vi "PH_PP_CurrentMeas.stop Task.vi"(0 "i ref in":refnum<vi>, 2 "Task #":i32, 5 "error in (no error)":errorcluster) -> (14 "i ref out":refnum<vi>, 19 "error out":errorcluster)   [LabVIEW 2014, in "PH_PP_CurrentMeas.lvlib"]
uses:
  PH_PP_CurrentMeas.lvlib
  PH_StatusHandler/PH_StatusHandler.Status.ctl
  PH_StatusHandler/PH_StatusHandler.lvlib
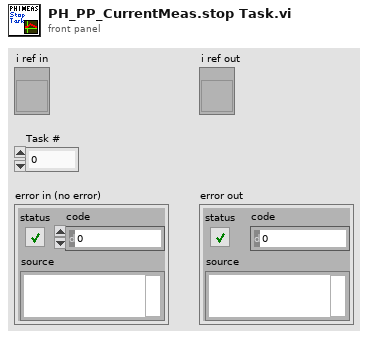
[diagram p1: front panel]
types:
  T1 = typedef "PH_PP_CurrentMeas.lvlib/PH_PP_CurrentMeas.i attribute.ctl" = cluster{"Status":cluster{"GUI Ref Hardware Feedback":refnum<vi>, "Tab Control":refnum<vi>}, "PU 1":cluster{"Instance":string, "Status":T2, "Ref Status ":refnum<vi>, "Data":waveform(dbl)[], "Ref Data":refnum<vi>}, "PU 2":cluster{"Instance":string, "Status":T2, "Ref Status ":refnum<vi>, "Data":waveform(dbl)[], "Ref Data":refnum<vi>}, "PU 3":cluster{"Instance":string, "Status":T2, "Ref Status ":refnum<vi>, "Data":waveform(dbl)[], "Ref Data":refnum<vi>}, "PU 4":cluster{"Instance":string, "Status":T2, "Ref Status ":refnum<vi>, "Data":waveform(dbl)[], "Ref Data":refnum<vi>}, "PU 5":cluster{"Instance":string, "Status":T2, "Ref Status ":refnum<vi>, "Data":waveform(dbl)[], "Ref Data":refnum<vi>}, "FR":cluster{"Instance":string, "Status":T2, "Ref Status ":refnum<vi>, "Data":waveform(dbl)[], "Ref Data":refnum<vi>}, "PA - 19mm 1":cluster{"Instance":string, "Status":T2, "Ref Status ":refnum<vi>}, "PA - 19mm 2":cluster{"Instance":string, "Status":T2, "Ref Status ":refnum<vi>, "no link":bool}, "PA - 45mm":cluster{"Instance":string, "Status":T2, "Ref Status ":refnum<vi>, "no link":bool}, "PA Data":cluster{"Data":waveform(dbl)[], "Ref":refnum<vi>}, "Sequencer":cluster{"Instance":string, "SM State Ref":refnum<vi>}, "Tasks":cluster{"Port":u16, "connection ID":refnum<k5>, "Status":T2, "Ref":refnum<vi>, "Ref Bar":refnum<vi>, "Feedback":cluster{"Received Data Sets":T3[], "Driver Error":errorcluster, "Connection not established":bool, "Error unpacking the data":bool, "No Task defined":bool, "Not triggered yet":bool}, "Data":waveform(dbl)[], "Ref Teststart Task":refnum<vi>}[], "in use":cluster{"MA DP":bool, "FR and PA":bool}, "DAQ Server":string}
  T2 = typedef "PH_StatusHandler.lvlib/PH_StatusHandler.Status.ctl" = i16
  T3 = typedef "PH_PP_CurrentMeas.lvlib/PH_PP_CurrentMeas.CommandCluster.ctl" = cluster{"Command":string, "Data":string, "error out":errorcluster}
  T4 = cluster{"Port":u16, "connection ID":refnum<k5>, "Status":T2, "Ref":refnum<vi>, "Ref Bar":refnum<vi>, "Feedback":cluster{"Received Data Sets":T3[], "Driver Error":errorcluster, "Connection not established":bool, "Error unpacking the data":bool, "No Task defined":bool, "Not triggered yet":bool}, "Data":waveform(dbl)[], "Ref Teststart Task":refnum<vi>}[]
  T5 = cluster{"Port":u16, "connection ID":refnum<k5>, "Status":T2, "Ref":refnum<vi>, "Ref Bar":refnum<vi>, "Feedback":cluster{"Received Data Sets":T3[], "Driver Error":errorcluster, "Connection not established":bool, "Error unpacking the data":bool, "No Task defined":bool, "Not triggered yet":bool}, "Data":waveform(dbl)[], "Ref Teststart Task":refnum<vi>}
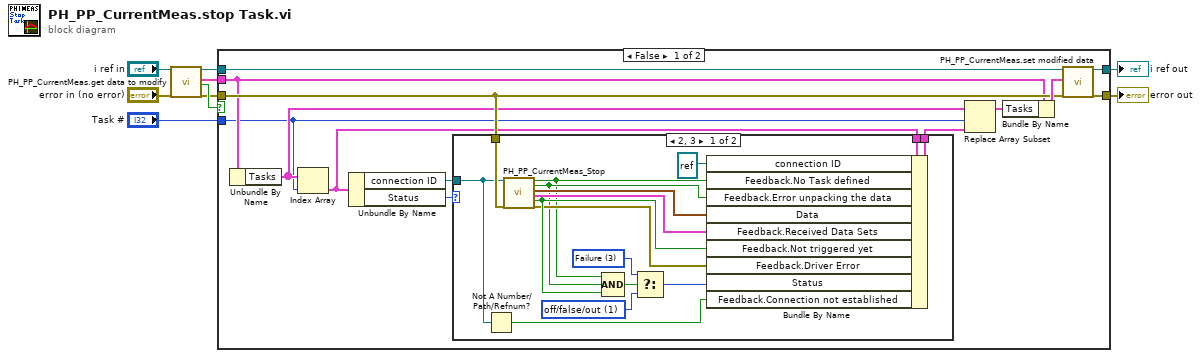
[diagram p0: block diagram]
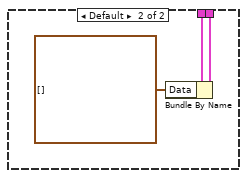
[diagram p2: hidden frame]
diagram:
  n1 = call "PH_PP_CurrentMeas.get data to modify.vi"("i ref in"="i ref in", "error in (no error)"="error in (no error)") -> ("i ref out"=w4:refnum<vi>, "i attribute"=w7:T1, "timed out"=w6:bool, "error out"=w5:errorcluster)  [unwired: 14 in]
  n2 = case shown="False" w6 {
    tunnel: w4 -> [w22 w43]
    tunnel: [w21 w43] -> w1
    tunnel: w5 -> [w16 w42]
    tunnel: [w20 w42] -> w2
    tunnel: w7 -> [w15 _]
    tunnel: "Task #" -> [w10 _]
    frame False {
      n3 = Unbundle By Name(w15) -> ("Tasks"=w11:T4)
      n4 = Index Array(array=w11, index=w10) -> (element=w14:T5)
      n5 = Unbundle By Name(w14) -> ("connection ID"=w13:refnum<k5>, "Status"=w12:T2)
      n6 = case shown="2, 3" w12 {
        tunnel: w14 -> [w38 w41]
        tunnel: [w37 w40] -> w17
        tunnel: w16 -> [w29 _]
        tunnel: w13 -> [w27 _]
        frame 2, 3 {
          w34 = T2 1 items=["no info", "off/false/out", "on/true/in", "Failure", "Alarm", "Status 1", "Status 2", "Status 3"] ("f")
          w35 = T2 3 items=["no info", "off/false/out", "on/true/in", "Failure", "Alarm", "Status 1", "Status 2", "Status 3"] ("Status")
          n7 = Not A Number/Path/Refnum?(number/path/refnum=w27) -> (NaN/Path/Refnum?=w26:bool)
          n8 = call "PH_PP_CurrentMeas_Stop.vi"("connection ID in"=w27, "error in (no error)"=w29) -> ("No Data achieved due to Task Failure"=w23:bool, "Error unpacking Data?"=w24:bool, "Measurement Data"=w25:waveform(dbl)[], "Receveived Data Sets"=w33:T3[], "No Data achieved due to no Trigger Signal"=w32:bool, "error out"=w31:errorcluster)  [unwired: 12 in]
          n9 = Compound Arithmetic op=AND(w23, w24, w32) -> (w36:bool)
          n10 = Select(t=w35, s=w36, f=w34) -> (s? t:f=w30:T2)
          n11 = Bundle By Name(cluster=w38, "connection ID"=refnum<k5> refnum, "Feedback.No Task defined"=w23, "Feedback.Error unpacking the data"=w24, "Data"=w25, "Feedback.Received Data Sets"=w33, "Feedback.Not triggered yet"=w32, "Feedback.Driver Error"=w31, "Status"=w30, "Feedback.Connection not established"=w26) -> (w37:T5)
        }
        frame Default {
          n12 = Bundle By Name(cluster=w41, "Data"=waveform(dbl)[] []) -> (w40:T5)
        }
      }
      n13 = Replace Array Subset(array=w11, new element=w17, index=w10) -> (w18:T4)
      n14 = Bundle By Name(cluster=w15, "Tasks"=w18) -> (w19:T1)
      n15 = call "PH_PP_CurrentMeas.set modified data.vi"("i ref in"=w22, "i attribute"=w19, "error in (no error)"=w16) -> ("i ref out"=w21:refnum<vi>, "error out"=w20:errorcluster)  [unwired: 15 in]
    }
    frame True {
    }
  }
  "error out" <- w2
  "i ref out" <- w1
